vi "TimestampFormat.vi"   [LabVIEW 2018, in "OXYGEN.lvlib"]
uses:
  OXYGEN.lvlib
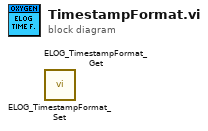
[diagram p0: block diagram]
diagram:
  n1 = call "ELOG_TimestampFormat_Set.vi"() -> ()  [unwired: 9 in, 3 out]
  n2 = call "ELOG_TimestampFormat_Get.vi"() -> ()  [unwired: 8 in, 4 out]
